vi "Constants.vi"   [LabVIEW 2020]
uses:
  Globals.vi
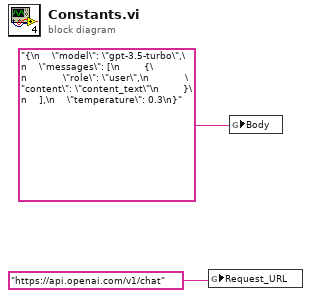
[diagram p0: block diagram]
diagram:
  n1 = global write "Globals.vi" "Request_URL"("https://api.openai.com/v1/chat" ("Path")) -> ()
  n2 = global write "Globals.vi" "Body"("{\n    \"model\": \"gpt-3.5-turbo\",\n    \"messages\": [\n        {\n            \"role\": \"user\",\n            \"content\": \"content_text\"\n        }\n    ],\n    \"temperature\": 0.3\n}" ("Request body")) -> ()
